vi "Get Image Data.vi"(11 "Image":T1) -> (0 "Image (RGBA)":u8[](array[numeric]), 1 "Channels":i32, 2 "Height":i32, 3 "Width":i32)   [LabVIEW 2020, in "G-Image.lvlib"]
doc: "Extract image data components from a LabVIEW image. The Image data will be converted from ARGB to RGBA memory layout."
uses:
  G-Image.lvlib
  <vilib>/picture/picture.llb/imagedata.ctl
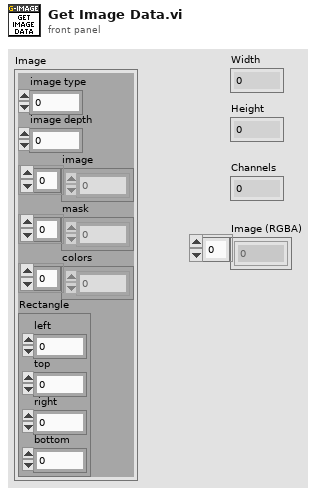
[diagram p1: front panel]
types:
  T1 = typedef "imagedata.ctl" = cluster{"image type":i32, "image depth":i32, "image":u8[], "mask":u8[], "colors":u32[], "Rectangle":cluster{"left":i16, "top":i16, "right":i16, "bottom":i16}}
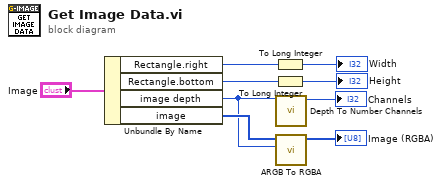
[diagram p0: block diagram]
diagram:
  n1 = Unbundle By Name("Image") -> ("Rectangle.right"=w9:i16, "Rectangle.bottom"=w8:i16, "image depth"=w2:i32, "image"=w7:u8[])
  n2 = To Long Integer(number=w9) -> (32bit integer=→"Width":i32)
  n3 = To Long Integer(number=w8) -> (32bit integer=→"Height":i32)
  n4 = call "Depth To Number Channels.vi"("Depth"=w2) -> ("Channels"=→"Channels":i32)  [unwired: 10 in]
  n5 = call "ARGB To RGBA.vi"("Depth"=w2, "ARGB"=w7) -> ("RGBA"=→"Image (RGBA)":u8[])  [unwired: 9 in]
